vi "Auto Diagnotics Run.vi"() -> ()   [LabVIEW 2012]
uses:
  Type/_GUI Method.ctl
  Type/_Lens Property.ctl
  Type/_Mass Range Property.ctl
  Type/_Mass Range Parameters.ctl
  Type/_RT Res Type.ctl
  Type/_Run Mode.ctl
  Type/_Run State.ctl
  Type/_RT Command.ctl
  Type/_Data Operation.ctl
  Type/_File Type.ctl
  Type/_Run Module.ctl
  Configuration/_Global Configuration.vi
  <vilib>/Utility/config.llb/Read Key (Path).vi
  <vilib>/Utility/file.llb/Read From Spreadsheet File (string).vi
  <vilib>/Utility/config.llb/Write Key (Path).vi
  <vilib>/Utility/config.llb/NI_LVConfig.lvlib
panel:
  out "GUI Method":T1={"Lenses"=[], "Mass Ranges"=[], "Acquire"=FALSE, "MCA"=FALSE, "Q1DC EN"=FALSE, "Q1 POL"=FALSE, "Q3 POL"=FALSE, "Q1 RF  EN"=FALSE, "Averaging"=FALSE, "Log Scale"=FALSE, "CPS"=FALSE, "Unit"=FALSE, "Data Path"=path "", "Run Mode"=enum."MRM (Q1/Q2)", "Fixed Mass (amu)"=1.0, "Q3DC EN"=FALSE, "Q3 RF  EN"=FALSE, "Negative"=FALSE} {"Mass Ranges"."Res" items=["High/High", "Medium/Medium", "Low/Low", "High/Medium", "High/Low", "Medium/High", "Medium/Low", "Low/High", "Low/Medium"]}
  in  "Run List":string[][](table)
  in  "Data Path:":path
  in  "Method Path:":path
  out "# of Samp":i32=1 caption="# of Samples"
  in  "Import":bool
  in  "Export":bool
  in  "Run":bool
  in  "Cancel":bool
  out "Run Time":i32=1 caption="Run Time (ms)"
  in  "Current Sample":i32=1 min=0
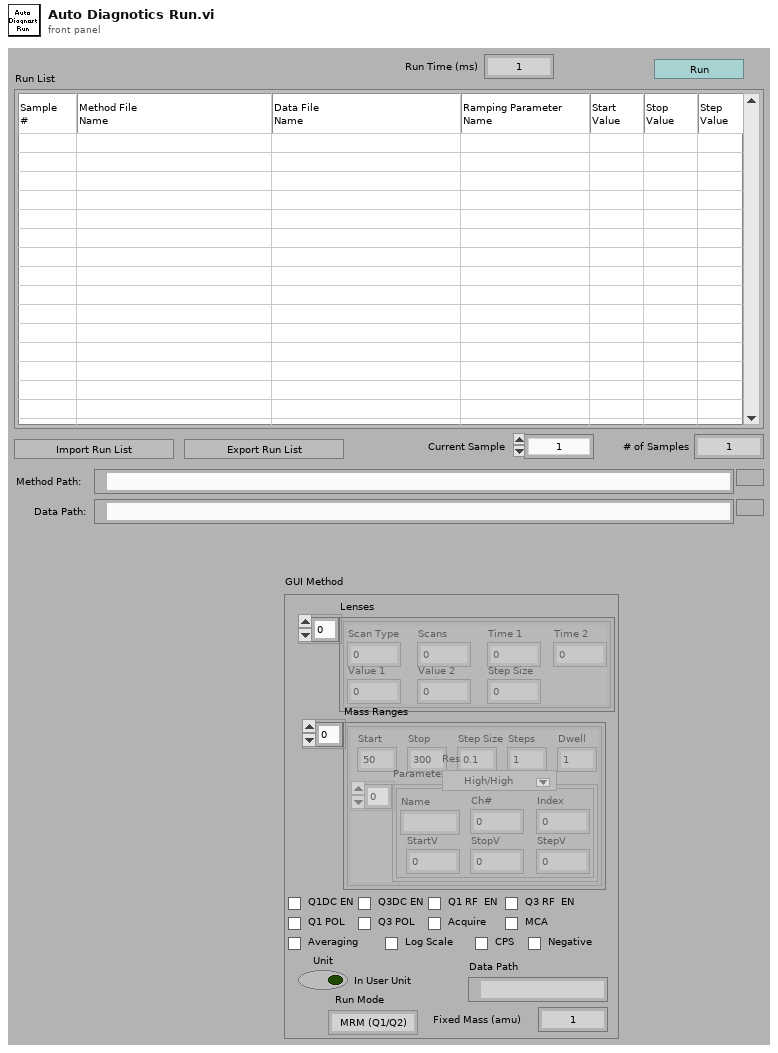
[diagram p1: front panel]
types:
  T1 = typedef "_GUI Method.ctl" = cluster{"Lenses":T2[], "Mass Ranges":T3[], "Acquire":bool, "MCA":bool, "Q1DC EN":bool, "Q1 POL":bool, "Q3 POL":bool, "Q1 RF  EN":bool, "Averaging":bool, "Log Scale":bool, "CPS":bool, "Unit":bool, "Data Path":path, "Run Mode":T6, "Fixed Mass (amu)":dbl, "Q3DC EN":bool, "Q3 RF  EN":bool, "Negative":bool}
  T2 = typedef "_Lens Property.ctl" = cluster{"Scan Type":u8, "Scans":i32, "Time 1":dbl, "Time 2":dbl, "Value 1":dbl, "Value 2":dbl, "Step Size":dbl}
  T3 = typedef "_Mass Range Property.ctl" = cluster{"Start":dbl, "Stop":dbl, "Step Size":dbl, "Steps":i32, "Dwell":dbl, "Parameters":T4[], "Res":T5}
  T4 = typedef "_Mass Range Parameters.ctl" = cluster{"Name":string, "Ch#":u8, "StartV":dbl, "StopV":dbl, "StepV":dbl, "Index":u8}
  T5 = typedef "_RT Res Type.ctl" = u16
  T6 = typedef "_Run Mode.ctl" = enum16{"MRM (Q1/Q2)", "Q1 Scan", "Q1 SRM", "Q2 Scan", "Q2 SRM", "Product Scan", "Precursor Scan", "Neutral Loss", "Neutral Gain"}
  T7 = typedef "_Run State.ctl" = enum16{"Init", "Update", "Start", "End", "Error"}
  T8 = typedef "_RT Command.ctl" = enum16{"Start", "Stop", "Runtime Update", "Get Data", "Get Info", "Get Status", "Get Param", "Get Config", "Get Table", "Read ADC", "Set Oscillator", "Update Config", "Update Table", "Set All Pol", "Set Pol and DC", "Set Max Mass", "Toggle RP", "Toggle EL", "Set PIC", "Initialize Turbo", "Send Turbo Comm", "Close Turbo", "P1", "P2", "P3", "Send Serial", "Set LC Out", "Get LC In", "Read VAC", "Test Table", "Toggle Power", "Get Startup", "Set Startup", "Get ADC Table", "Set ADC Table", "Get Brief Status", "Get Detail Status", "Auxiliary Update", "Set CC Logics", "Set CC Input Logics", "Ignore Error"}
  T9 = typedef "_Data Operation.ctl" = enum8{"Initialize", "Get Data", "Set Data", "Close"}
  T10 = typedef "_File Type.ctl" = enum16{"Configuration", "Old Configuration", "Calibration", "Resolution", "Diagnostic Method", "Old Method", "Acq Method", "Samp List"}
  T11 = enum32{"Bad", "Idle", "Run top level", "Running"}
  T12 = enum32{"existing file", "new file", "new or existing file", "existing dir", "new dir", "new or existing dir", "existing file (use LLBs)", "new file (use LLBs)", "new or existing file (use LLBs)", "new or existing file or directory (use LLBs)"}
  T13 = enum8{"Enabled", "Disabled", "Disabled and Grayed Out"}
  T14 = typedef "NI_LVConfig.lvlib/Config Data RefNum.ctl" = refnum<k1>
  T15 = cluster{"Update":bool, "Running":bool, "Run List":string[][]}
  T16 = typedef "_RT Configuration 2.ctl" = cluster{"Name":string, "Ch#":u8, "Min":dbl, "Max":dbl, "Def+":dbl, "Def-":dbl, "Offset":dbl, "Slope":dbl, "Type":u8, "Description":string, "SettleT":dbl}
  T17 = typedef "_Run Module.ctl" = u16
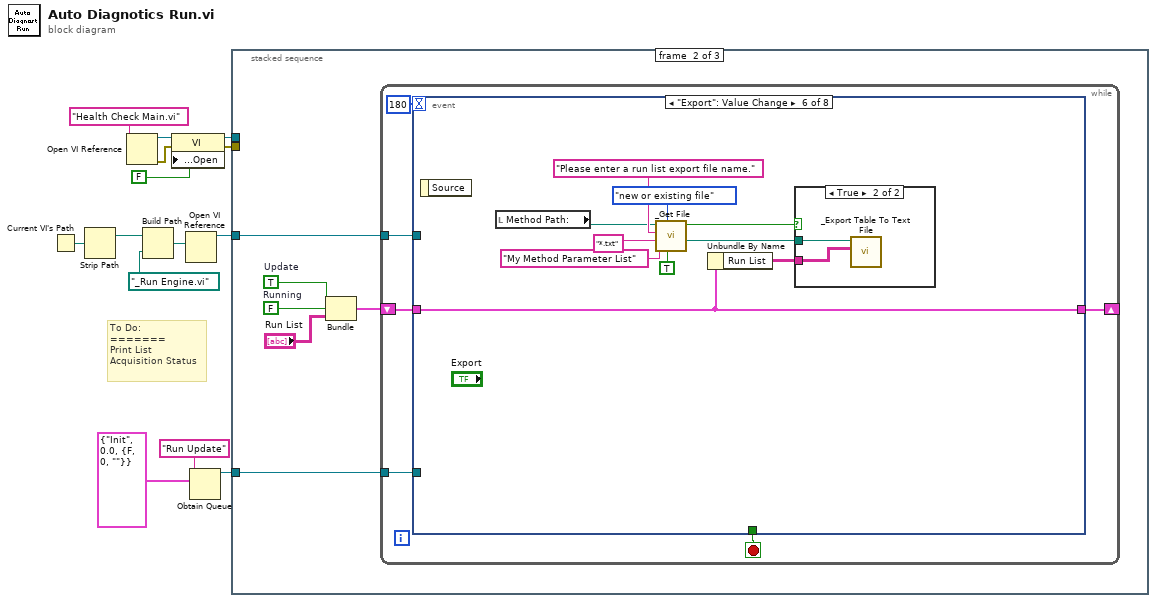
[diagram p0: block diagram]
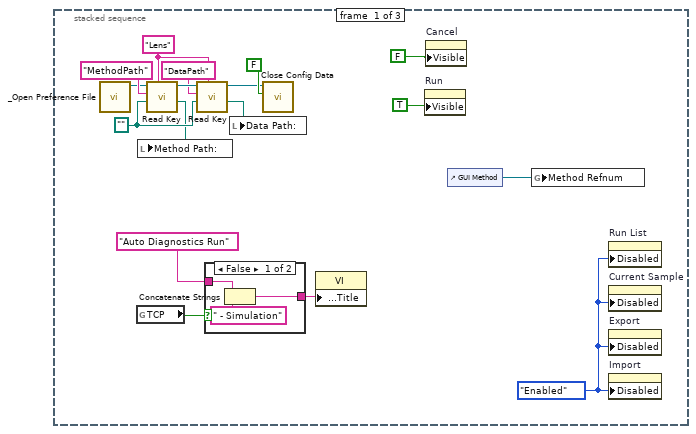
[diagram p2: hidden frame]
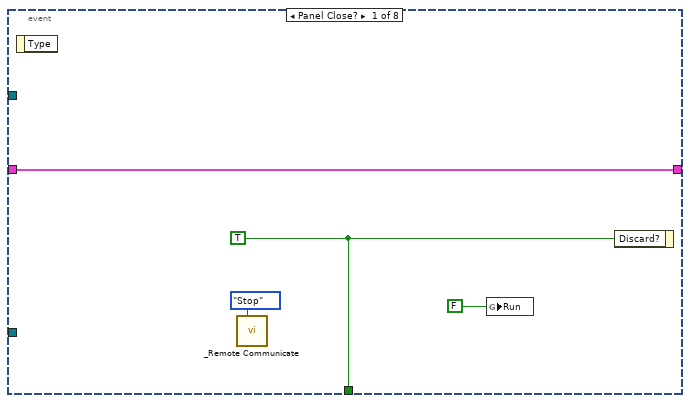
[diagram p4: hidden frame]
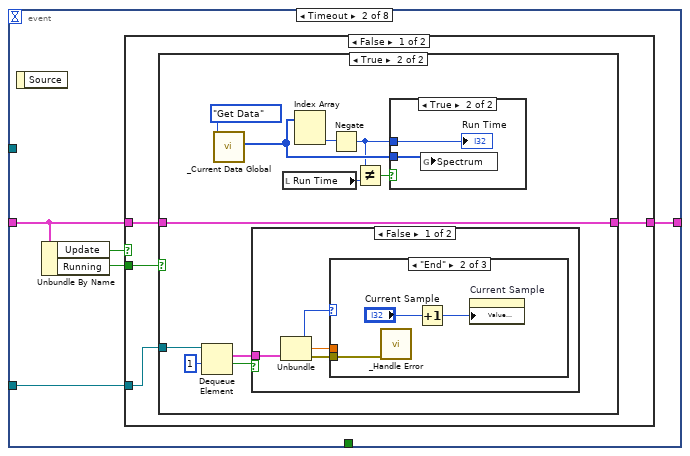
[diagram p5: hidden frame]
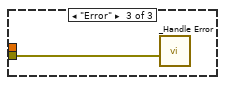
[diagram p9: hidden frame]
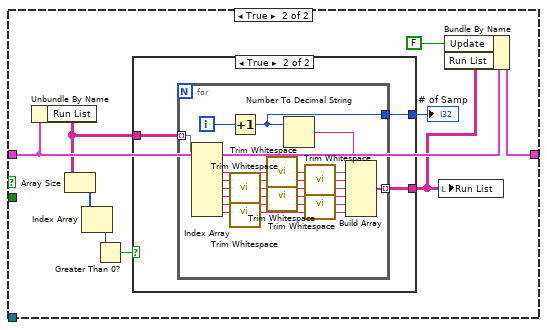
[diagram p11: hidden frame]
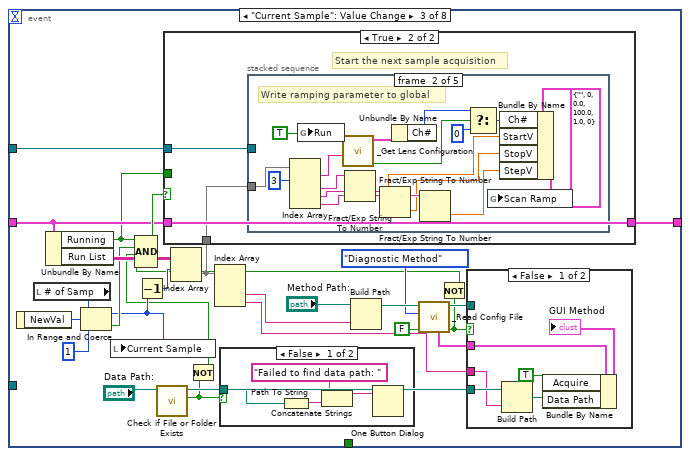
[diagram p13: hidden frame]
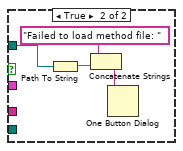
[diagram p15: hidden frame]
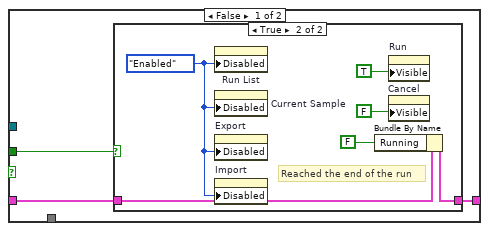
[diagram p16: hidden frame]
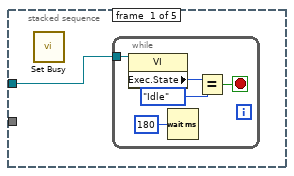
[diagram p18: hidden frame]
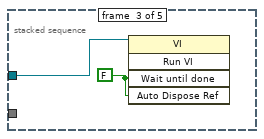
[diagram p19: hidden frame]
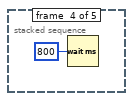
[diagram p20: hidden frame]
diagram:
  # "To Do:\n=======\nPrint List\nAcquisition Status"
  n1 = Current VI's Path() -> (path=w11:path)
  n2 = Strip Path(path=w11) -> (stripped path=w7:path)  [unwired: 1 out]
  n3 = Open VI Reference(vi path="Health Check Main.vi") -> (vi reference=w5:refnum<vi>, error out=w4:errorcluster)  [unwired: 1 in, 4 out]
  n4 = Build Path(base path=w7, name or relative path=path "_Run Engine.vi") -> (appended path=w9:path)
  n5 = property class="VI"(reference=w5, error in=w4, "Front Panel Window:Open"=FALSE) -> (reference out=w2:refnum<vi>, error out=w1:errorcluster)
  n6 = Open VI Reference(vi path=w9) -> (vi reference=w8:refnum<vi>)  [unwired: 1 in, 5 out]
  n7 = Obtain Queue(name (unnamed)="Run Update", element data type=cluster{T7, dbl, "error out":errorcluster} {enum."Init", 0.0, "error out"={"status"=FALSE, "code"=0, "source"=""}}) -> (queue out=w12:refnum<queue>)  [unwired: 3 in, 2 out]
  n8 = stacked-sequence {
    tunnel: w12 -> [_ w41 w272]
    tunnel: w8 -> [_ w40 w271]
    tunnel: w2 -> [_ _ w267]
    tunnel: w1 -> [_ _ w266]
    frame #0 {
      w16 = T13."Enabled" ("Disabled")
      w22 = "Lens" ("section")
      w20 = path ""
      n9 = call "_Open Preference File.vi"() -> ("refnum"=w24:T14)  [unwired: 1 in, 6 out]
      n10 = global read "_Global Configuration.vi" "TCP"() -> (w29:bool)
      n11 = call-poly <vilib>:"Read Key.vi"("section"=w22, "default value"=w20, "key"="MethodPath", "refnum"=w24) -> ("value"=w19:path, "refnum out"=w23:T14)  [unwired: 1 in, 5 out]
      n12 = local write "Method Path:"(w19) -> ()
      n13 = call-poly <vilib>:"Read Key.vi"("section"=w22, "default value"=w20, "key"="DataPath", "refnum"=w23) -> ("value"=w17:path, "refnum out"=w18:T14)  [unwired: 1 in, 5 out]
      n14 = case shown="False" w29 {
        tunnel: "Auto Diagnostics Run" ("string") -> [w34 w35]
        tunnel: [w32 w35] -> w30
        frame False {
          n15 = Concatenate Strings(w34, " - Simulation" ("string")) -> (w32:string)
        }
        frame True {
        }
      }
      n16 = local write "Data Path:"(w17) -> ()
      n17 = call <vilib>:"Close Config Data.vi"("write file if changed (T)"=FALSE ("write configuration file? (F)"), "refnum"=w18) -> ()  [unwired: 1 in, 9 out]
      n18 = property class="VI"("Front Panel Window:Title"=w30) -> ()  [unwired: 2 in, 2 out]
      n19 = property on="Run" class="Bool"("Visible"=TRUE) -> ()  [unwired: 2 in, 2 out]
      n20 = property on="Cancel" class="Bool"("Visible"=FALSE ("Unit")) -> ()  [unwired: 2 in, 2 out]
      n21 = control-ref of="GUI Method"() -> (w15:refnum<vi>)
      n22 = global write "_Global Configuration.vi" "Method Refnum"(w15) -> ()
      n23 = property on="Run List" class="Tbl (strict)"("Disabled"=w16) -> ()  [unwired: 2 in, 2 out]
      n24 = property on="Current Sample" class="DigNum (strict)"("Disabled"=w16) -> ()  [unwired: 2 in, 2 out]
      n25 = property on="Export" class="Bool"("Disabled"=w16) -> ()  [unwired: 2 in, 2 out]
      n26 = property on="Import" class="Bool"("Disabled"=w16) -> ()  [unwired: 2 in, 2 out]
    }
    frame #1 {
      w38 = FALSE  # Running
      w39 = TRUE  # Update
      n27 = Bundle("Update"=w39, "Running"=w38, "Run List"="Run List") -> (w37:T15)  [unwired: 1 out]
      n28 = while {
        shift-right: [w44] -> _
        shift-left: w37 -> [w46]
        tunnel: w41 -> [w43]
        tunnel: w40 -> [w42]
        stop <- w47 stop-if-true
        n29 = event shown="[5] \"Export\": Value Change" {
          selector: _ -> [_ _ _ _ _ _ _ _]
          dyn-events: _ -> [_ _ _ _ _ _ _ _]
          timeout: 180 -> [_ _ _ _ _ _ _ _]
          tunnel: [w48 _ _ _ _ _ _ _] -> w47
          tunnel: w46 -> [w49 w54 w133 w195 w210 w216 w229 w242]
          tunnel: [w49 w56 w132 w194 w209 w216 w235 w238] -> w44
          tunnel: w43 -> [_ w55 _ _ _ _ w237 _]
          tunnel: w42 -> [_ _ w134 _ _ _ _ w241]
          event Panel Close? {
            w48 = TRUE ("Discard?")
            n30 = event-data() -> ()  [unwired: 2 out]
            n31 = call "_Remote Communicate.vi"("Command"=_RT_Command."Stop") -> ()  [unwired: 5 in, 4 out]
            n32 = global write "_Global Configuration.vi" "Run"(FALSE ("Update")) -> ()
            n33 = event-data("Discard?"=w48) -> ()  [unwired: 1 in, 1 out]
          }
          event Timeout {
            n34 = event-data() -> ()  [unwired: 2 out]
            n35 = Unbundle By Name(w54) -> ("Update"=w53:bool, "Running"=w52:bool)
            n36 = case shown="False" w53 {
              tunnel: w54 -> [w58 w91]
              tunnel: [w57 w89] -> w56
              tunnel: w52 -> [w60 _]
              tunnel: w55 -> [w59 _]
              frame False {
                n37 = case shown="True" w60 {
                  tunnel: w59 -> [_ w72]
                  tunnel: w58 -> [w61 w62]
                  tunnel: [w61 w62] -> w57
                  frame False {
                  }
                  frame True {
                    n38 = Dequeue Element(queue=w72, timeout in ms (-1)=1) -> (element=w70:cluster{T7, dbl, "error out":errorcluster}, timed out?=w69:bool)  [unwired: 1 in, 2 out]
                    n39 = call "_Current Data Global.vi"("Operation"=_Data_Operation."Get Data") -> ("Latest Raw Data"=w65:i32[])  [unwired: 3 in, 3 out]
                    n40 = case shown="False" w69 {
                      tunnel: w70 -> [w78 _]
                      frame False {
                        n41 = Unbundle(w78) -> (w77:T7, w75:dbl, "error out"=w76:errorcluster)
                        n42 = case shown="\"End\"" w77 {
                          tunnel: w76 -> [_ w81 w82]
                          tunnel: w75 -> [_ _ _]
                          frame "Init", Default {
                          }
                          frame "End" {
                            n43 = call "_Handle Error.vi"("error in (no error)"=w81) -> ()  [unwired: 2 in, 5 out]
                            n44 = Increment(x="Current Sample") -> (x+1=w80:i32)
                            n45 = property on="Current Sample" class="DigNum (strict)"("Value (Signaling)"=w80) -> ()  [unwired: 2 in, 2 out]
                          }
                          frame "Error" {
                            n46 = call "_Handle Error.vi"("error in (no error)"=w82) -> ()  [unwired: 2 in, 5 out]
                          }
                        }
                      }
                      frame True {
                      }
                    }
                    n47 = local read "Run Time"() -> (w67:i32)
                    n48 = Index Array(array=w65) -> (element #2=w64:i32)  [unwired: 2 in, 1 out]
                    n49 = Negate(x=w64) -> (-x=w63:i32)
                    n50 = Not Equal?(x=w63, y=w67) -> (x != y?=w66:bool)
                    n51 = case shown="True" w66 {
                      tunnel: w65 -> [_ w73]
                      tunnel: w63 -> [_ w74]
                      frame False {
                      }
                      frame True {
                        n52 = global write "_Global Configuration.vi" "Spectrum"(w73) -> ()
                        "Run Time" <- w74
                      }
                    }
                  }
                }
              }
              frame True {
                n53 = Unbundle By Name(w91) -> ("Run List"=w87:string[][])
                n54 = Array Size(array=w87) -> (size(s)=w86:i32[])
                n55 = Index Array(array=w86) -> (element=w85:i32)  [unwired: 1 in]
                n56 = Greater Than 0?(x=w85) -> (x > 0?=w84:bool)
                n57 = case shown="True" w84 {
                  tunnel: [_ w94] -> w88
                  tunnel: [_ w93] -> w83
                  tunnel: w87 -> [_ w92]
                  frame False {
                  }
                  frame True {
                    n58 = for {
                      tunnel: w92 -> [w111] mode=indexing
                      tunnel: [w109] -> w94
                      tunnel: [w107] -> w93 mode=indexing
                      i -> [w110]
                      n59 = Index Array(array=w111) -> (element #2=w106:string, element #3=w105:string, element #4=w102:string, element #5=w100:string, element #6=w99:string, element #7=w96:string)  [unwired: 7 in, 1 out]
                      n60 = Increment(x=w110) -> (x+1=w109:i32)
                      n61 = call <vilib>:"Trim Whitespace.vi"("string"=w102) -> ("trimmed string"=w101:string)  [unwired: 1 in]
                      n62 = call <vilib>:"Trim Whitespace.vi"("string"=w96) -> ("trimmed string"=w95:string)  [unwired: 1 in]
                      n63 = call <vilib>:"Trim Whitespace.vi"("string"=w106) -> ("trimmed string"=w104:string)  [unwired: 1 in]
                      n64 = call <vilib>:"Trim Whitespace.vi"("string"=w100) -> ("trimmed string"=w98:string)  [unwired: 1 in]
                      n65 = Number To Decimal String(number=w109) -> (decimal integer string=w108:string)  [unwired: 1 out]
                      n66 = call <vilib>:"Trim Whitespace.vi"("string"=w105) -> ("trimmed string"=w103:string)  [unwired: 1 in]
                      n67 = call <vilib>:"Trim Whitespace.vi"("string"=w99) -> ("trimmed string"=w97:string)  [unwired: 1 in]
                      n68 = Build Array(w108, w104, w103, w101, w98, w97, w95) -> (w107:string[])
                    }
                  }
                }
                "# of Samp" <- w88
                n69 = local write "Run List"(w83) -> ()
                n70 = Bundle By Name(cluster=w91, "Update"=FALSE, "Run List"=w83) -> (w89:T15)
              }
            }
          }
          event "Current Sample": Value Change {
            n71 = event-data() -> ("NewVal"=w129:i32)  [unwired: 1 out]
            n72 = local read "# of Samp"() -> (w128:i32)
            n73 = Unbundle By Name(w133) -> ("Running"=w131:bool, "Run List"=w137:string[][])
            n74 = In Range and Coerce(upper limit=w128, x=w129, lower limit=1) -> (coerced(x)=w130:i32, In Range?=w136:bool)
            n75 = local write "Current Sample"(w130) -> ()
            n76 = Decrement(x=w130) -> (x-1=w127:i32)
            n77 = call <vilib>:"Check if File or Folder Exists.vi"("path"="Data Path:") -> ("file or folder exists?"=w115:bool, "dup path"=w118:path)  [unwired: 8 in, 1 out]
            n78 = Index Array(array=w137, index (row)=w127) -> (element=w116:string[])  [unwired: 1 in]
            n79 = Not(x=w115) -> (.not. x?=w114:bool)
            n80 = Index Array(array=w116) -> (element #2=w125:string, element #3=w117:string)  [unwired: 3 in, 1 out]
            n81 = case shown="False" w115 {
              tunnel: w118 -> [w140 _]
              frame False {
                n82 = Path To String(path=w140) -> (string=w142:string)
                n83 = Concatenate Strings("Failed to find data path: ", w142) -> (w139:string)
                n84 = One Button Dialog(message=w139) -> ()  [unwired: 1 in, 1 out]
              }
              frame True {
              }
            }
            n85 = Build Path(base path="Method Path:", name or relative path=w125) -> (appended path=w123:path)
            n86 = call "_Read Config File.vi"("advisory dialog? (display:T)"=FALSE, "File Type (config)"=_File_Type."Diagnostic Method", "start path  (Not A Path)"=w123) -> ("error"=w113:bool, "new file path"=w119:path, "GUI Method"=w120:T1)  [unwired: 6 out]
            n87 = Not(x=w113) -> (.not. x?=w112:bool)
            n88 = Compound Arithmetic op=AND(w131, w136, w114, w112) -> (w135:bool)
            n89 = case shown="True" w135 {
              tunnel: w134 -> [_ w165]
              tunnel: w133 -> [w155 w164]
              tunnel: [w154 w164] -> w132
              tunnel: w131 -> [w153 _]
              tunnel: w116 -> [_ w163]
              frame False {
                n90 = case shown="True" w153 {
                  tunnel: w155 -> [w156 w162]
                  tunnel: [w156 w161] -> w154
                  frame False {
                  }
                  frame True {
                    w157 = T13."Enabled" ("Disabled")
                    # "Reached the end of the run"
                    n91 = property on="Run List" class="Tbl (strict)"("Disabled"=w157) -> ()  [unwired: 2 in, 2 out]
                    n92 = property on="Current Sample" class="DigNum (strict)"("Disabled"=w157) -> ()  [unwired: 2 in, 2 out]
                    n93 = property on="Export" class="Bool"("Disabled"=w157) -> ()  [unwired: 2 in, 2 out]
                    n94 = property on="Import" class="Bool"("Disabled"=w157) -> ()  [unwired: 2 in, 2 out]
                    n95 = Bundle By Name(cluster=w162, "Running"=FALSE) -> (w161:T15)
                    n96 = property on="Run" class="Bool"("Visible"=TRUE) -> ()  [unwired: 2 in, 2 out]
                    n97 = property on="Cancel" class="Bool"("Visible"=FALSE) -> ()  [unwired: 2 in, 2 out]
                  }
                }
              }
              frame True {
                # "Start the next sample acquisition"
                n98 = stacked-sequence {
                  tunnel: w165 -> [w166 _ w189 _ _]
                  tunnel: w163 -> [_ w187 _ _ _]
                  frame #0 {
                    n99 = call <vilib>:"Set Busy.vi"() -> ()  [unwired: 4 in, 8 out]
                    n100 = while {
                      tunnel: w166 -> [w171]
                      stop <- w168 stop-if-true
                      n101 = property class="VI"(reference=w171) -> ("Exec.State"=w170:T11)  [unwired: 1 in, 2 out]
                      n102 = Wait (ms)(milliseconds to wait=u32 180) -> ()  [unwired: 1 out]
                      n103 = Equal?(x=w170, y=T11."Idle") -> (x = y?=w168:bool)
                    }
                  }
                  frame #1 {
                    # "Write ramping parameter to global"
                    n104 = Index Array(array=w187, index #1=3 ("index")) -> (element #1=w184:string, element #2=w183:string, element #3=w182:string, element #4=w181:string)  [unwired: 3 in]
                    n105 = global write "_Global Configuration.vi" "Run"(TRUE ("Update")) -> ()
                    n106 = call "_Get Lens Configuration.vi"("Name"=w184) -> ("Found"=w179:bool, "Lens Configuration"=w185:T16)  [unwired: 1 in, 4 out]
                    n107 = Fract/Exp String To Number(string=w183) -> (number=w175:dbl)  [unwired: 3 in, 1 out]
                    n108 = Fract/Exp String To Number(string=w182) -> (number=w174:dbl)  [unwired: 3 in, 1 out]
                    n109 = Unbundle By Name(w185) -> ("Ch#"=w178:u8)
                    n110 = Fract/Exp String To Number(string=w181) -> (number=w173:dbl)  [unwired: 3 in, 1 out]
                    n111 = Select(t=w178, s=w179, f=u8 0) -> (s? t:f=w176:u8)
                    n112 = Bundle By Name(cluster=T4 {"Name"="", "Ch#"=0, "StartV"=0.0, "StopV"=100.0, "StepV"=1.0, "Index"=0} ("MR Parameters"), "Ch#"=w176, "StartV"=w175, "StopV"=w174, "StepV"=w173) -> (w172:T4)
                    n113 = global write "_Global Configuration.vi" "Scan Ramp"(w172) -> ()
                  }
                  frame #2 {
                    w190 = FALSE ("Wait until done")
                    n114 = invoke class="VI" method="Run VI"(reference=w189, "Wait until done"=w190, "Auto Dispose Ref"=w190) -> ()  [unwired: 2 in, 5 out]
                  }
                  frame #3 {
                    n115 = Wait (ms)(milliseconds to wait=u32 800) -> ()  [unwired: 1 out]
                  }
                  frame #4 {
                    n116 = call <vilib>:"Unset Busy.vi"() -> ()  [unwired: 2 in, 10 out]
                  }
                }
              }
            }
            n117 = case shown="False" w113 {
              tunnel: w120 -> [w148 _]
              tunnel: w119 -> [_ w149]
              tunnel: w118 -> [w146 _]
              tunnel: w117 -> [w145 _]
              frame False {
                n118 = Build Path(base path=w146, name or relative path=w145) -> (appended path=w144:path)
                n119 = Bundle By Name(cluster=w148, "Acquire"=TRUE, "Data Path"=w144) -> (→"GUI Method":T1)
              }
              frame True {
                n120 = Path To String(path=w149) -> (string=w150:string)
                n121 = Concatenate Strings("Failed to load method file: ", w150) -> (w152:string)
                n122 = One Button Dialog(message=w152) -> ()  [unwired: 1 in, 1 out]
              }
            }
          }
          event "Run List": Value Change {
            n123 = event-data() -> ("NewVal"=w193:string[][])  [unwired: 1 out]
            n124 = Bundle By Name(cluster=w195, "Update"=TRUE, "Run List"=w193) -> (w194:T15)
          }
          event "Import": Value Change {
            n125 = event-data() -> ()  [unwired: 2 out]
            n126 = Unbundle By Name(w210) -> ("Update"=w198:bool, "Run List"=w201:string[][])
            n127 = local read "Method Path:"() -> (w202:path)
            n128 = call "_Get File.vi"("For Write (T)"=FALSE, "select mode (new or existing)"=T12."existing file", "extension (isd)"="*.txt" ("pattern (all files)"), "prompt"="Please select a run list import file name.", "Start Path"=w202) -> ("Seleted File"=w200:path, "Exists"=w208:bool, "Succeeded"=w207:bool)  [unwired: 1 in, 1 out]
            n129 = And(x=w207, y=w208) -> (x .and. y?=w197:bool)
            n130 = case shown="True" w197 {
              selector: w197 -> [_ w213]
              tunnel: w201 -> [w212 _]
              tunnel: w200 -> [_ w215]
              tunnel: [w212 w214] -> w199
              tunnel: w198 -> [w211 _]
              tunnel: [w211 w213] -> w196
              frame False {
              }
              frame True {
                n131 = call-poly <vilib>:"Read From Spreadsheet File.vi"("file path (dialog if empty)"=w215) -> ("all rows"=w214:string[][])  [unwired: 6 in, 4 out]
              }
            }
            n132 = Bundle By Name(cluster=w210, "Update"=w196, "Run List"=w199) -> (w209:T15)
          }
          event "Export": Value Change {
            n133 = event-data() -> ()  [unwired: 2 out]
            n134 = local read "Method Path:"() -> (w220:path)
            n135 = call "_Get File.vi"("For Write (T)"=TRUE, "select mode (new or existing)"=T12."new or existing file", "default name"="My Method Parameter List", "extension (isd)"="*.txt" ("pattern (all files)"), "prompt"="Please enter a run list export file name.", "Start Path"=w220) -> ("Seleted File"=w218:path, "Succeeded"=w219:bool)  [unwired: 2 out]
            n136 = Unbundle By Name(w216) -> ("Run List"=w217:string[][])
            n137 = case shown="True" w219 {
              tunnel: w218 -> [_ w227]
              tunnel: w217 -> [_ w226]
              frame False {
              }
              frame True {
                n138 = call "_Export Table To Text File.vi"("2D data"=w226, "file path (dialog if empty)"=w227) -> ()  [unwired: 4 in, 3 out]
              }
            }
          }
          event "Run": Value Change {
            w228 = T13."Disabled" ("Disabled")
            w232 = T17 1 items=["Diagnostics", "Tune", "Acquisition"] ("RunModule")
            n139 = event-data() -> ()  [unwired: 2 out]
            n140 = Flush Queue(queue=w237) -> ()  [unwired: 1 in, 3 out]
            n141 = global write "_Global Configuration.vi" "RunModule"(w232) -> ()
            n142 = property on="Current Sample" class="DigNum (strict)"("Value (Signaling)"=1) -> ()  [unwired: 2 in, 2 out]
            n143 = property on="Run" class="Bool"("Visible"=FALSE) -> ()  [unwired: 2 in, 2 out]
            n144 = property on="Cancel" class="Bool"("Visible"=TRUE) -> ()  [unwired: 2 in, 2 out]
            n145 = property on="Run List" class="Tbl (strict)"("Disabled"=w228) -> ()  [unwired: 2 in, 2 out]
            n146 = property on="Current Sample" class="DigNum (strict)"("Disabled"=w228) -> ()  [unwired: 2 in, 2 out]
            n147 = property on="Export" class="Bool"("Disabled"=w228) -> ()  [unwired: 2 in, 2 out]
            n148 = property on="Import" class="Bool"("Disabled"=w228) -> ()  [unwired: 2 in, 2 out]
            n149 = call "_Launch Dynamic VI.vi"("VI Name"=path "Real Time Display.vi" ("name or relative path")) -> ()  [unwired: 4 out]
            n150 = Bundle By Name(cluster=w229, "Running"=TRUE) -> (w235:T15)
          }
          event "Cancel": Value Change {
            n151 = event-data() -> ()  [unwired: 7 out]
            n152 = stacked-sequence {
              tunnel: w242 -> [_ w245 _]
              tunnel: [_ w245 _] -> w239
              tunnel: w241 -> [_ w244 _]
              frame #0 {
                n153 = call <vilib>:"Set Busy.vi"() -> ()  [unwired: 4 in, 8 out]
                n154 = global write "_Global Configuration.vi" "Run"(FALSE ("Update")) -> ()
              }
              frame #1 {
                n155 = while {
                  tunnel: w244 -> [w250]
                  stop <- w247 stop-if-true
                  n156 = property class="VI"(reference=w250) -> ("Exec.State"=w249:T11)  [unwired: 1 in, 2 out]
                  n157 = Wait (ms)(milliseconds to wait=u32 180) -> ()  [unwired: 1 out]
                  n158 = Equal?(x=w249, y=T11."Idle") -> (x = y?=w247:bool)
                }
              }
              frame #2 {
                w251 = T13."Enabled" ("Disabled")
                n159 = call <vilib>:"Unset Busy.vi"() -> ()  [unwired: 2 in, 10 out]
                n160 = property on="Run" class="Bool"("Visible"=TRUE) -> ()  [unwired: 2 in, 2 out]
                n161 = property on="Cancel" class="Bool"("Visible"=FALSE) -> ()  [unwired: 2 in, 2 out]
                n162 = call "_Remote Wait Until Done.vi"() -> ("error out"=w252:errorcluster)  [unwired: 2 in, 1 out]
                n163 = call "_Remote Park Lens.vi"("error in"=w252) -> ()  [unwired: 1 in, 6 out]
                n164 = property on="Run List" class="Tbl (strict)"("Disabled"=w251) -> ()  [unwired: 2 in, 2 out]
                n165 = property on="Current Sample" class="DigNum (strict)"("Disabled"=w251) -> ()  [unwired: 2 in, 2 out]
                n166 = property on="Export" class="Bool"("Disabled"=w251) -> ()  [unwired: 2 in, 2 out]
                n167 = property on="Import" class="Bool"("Disabled"=w251) -> ()  [unwired: 2 in, 2 out]
              }
            }
            n168 = Bundle By Name(cluster=w239, "Running"=FALSE) -> (w238:T15)
          }
        }
      }
    }
    frame #2 {
      w262 = "Lens" ("section")
      n169 = property class="VI"(reference=w267, error in=w266, "Front Panel Window:Open"=TRUE) -> (reference out=w268:refnum<vi>, error out=w269:errorcluster)
      n170 = Close Reference(reference=w271) -> ()  [unwired: 1 in, 1 out]
      n171 = Release Queue(queue=w272) -> ()  [unwired: 1 in, 4 out]
      n172 = Close Reference(reference=w268, error in (no error)=w269) -> ()  [unwired: 1 out]
      n173 = local read "Method Path:"() -> (w259:path)
      n174 = local read "Data Path:"() -> (w255:path)
      n175 = call "_Open Preference File.vi"() -> ("error"=w258:errorcluster, "refnum"=w264:T14)  [unwired: 1 in, 5 out]
      n176 = call-poly <vilib>:"Write Key.vi"("section"=w262, "error in (no error)"=w258, "value"=w259, "key"="MethodPath", "refnum"=w264) -> ("error out"=w257:errorcluster, "refnum out"=w263:T14)  [unwired: 4 in, 1 out]
      n177 = call-poly <vilib>:"Write Key.vi"("section"=w262, "error in (no error)"=w257, "value"=w255, "key"="DataPath", "refnum"=w263) -> ("error out"=w256:errorcluster, "refnum out"=w260:T14)  [unwired: 4 in, 1 out]
      n178 = call <vilib>:"Close Config Data.vi"("error in (no error)"=w256, "refnum"=w260) -> ()  [unwired: 1 in, 9 out]
    }
  }
